vi "Add Error Core.vi"(8 "error in (no error)":errorcluster, 10 "String to Append":string, 11 "Error":T1) -> (0 "error out":errorcluster)   [LabVIEW 2021, in "CIFCoreCommon.lvlib"]
uses:
  CIFCoreCommon.lvlib
  <vilib>/CIF Foundation/CIF Utilities/Errors/Errors_CIF_U.lvlib
  Typedef/Errors.ctl
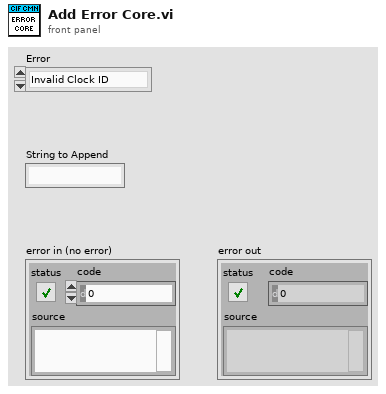
[diagram p1: front panel]
types:
  T1 = typedef "CIFCoreCommon.lvlib/Errors.ctl" = enum16{"Invalid Clock ID", "Long Sleep", "gRPC Server Not Found", "Config Parse", "Timestamp Wrap", "Delayed Execution", "Duplicate Channel", "Missing Channel", "Incorrect Type", "Flatten Error", "Unflatten Data", "Unique Name", "Plugin Not Found", "Plugin Type Not Found", "Plugin Version Not Found", "Manager Not Found", "Numerical Issue", "Time Jump", "Clock ID Match", "Channel Length", "Plugin Connection", "gRPC Server Connection", "PPL Name Match", "Build", "Config Log Parse", "Plugin Load", "UI Subpanel Load", "Python Name", "Invalid Name", "Unable to Change Ch Buffer", "Failed Kill", "Failed SysExec", "Function Not Implemented", "Load Timeout", "Invalid FTE", "Manager Crash"}
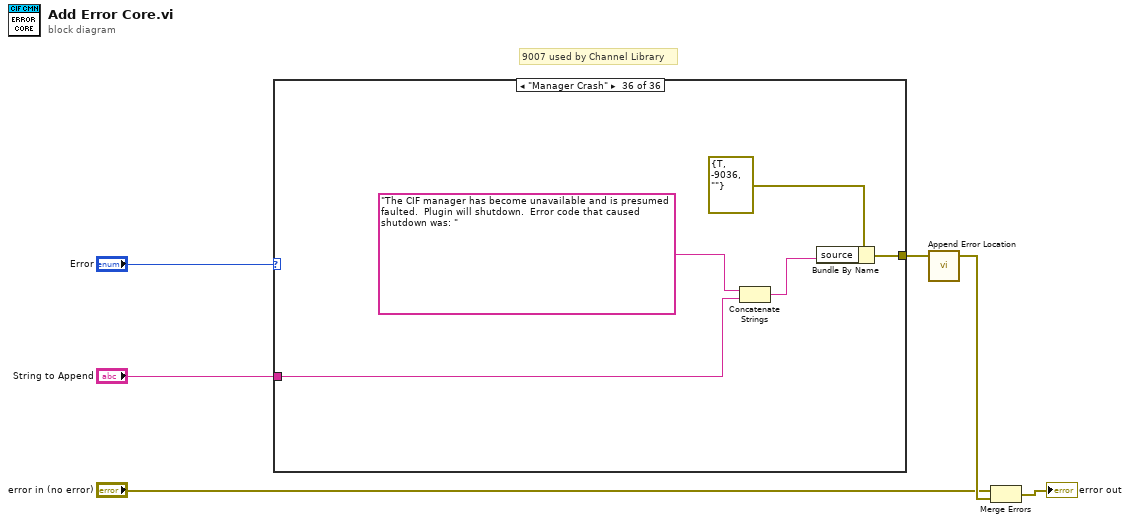
[diagram p0: block diagram]
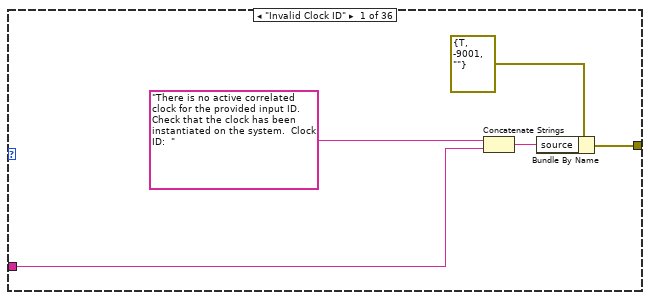
[diagram p2: hidden frame]
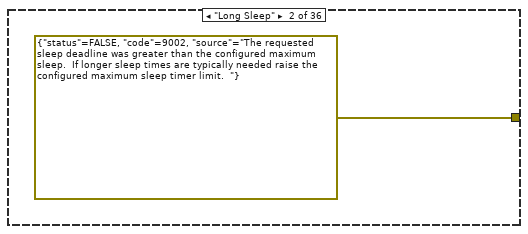
[diagram p3: hidden frame]
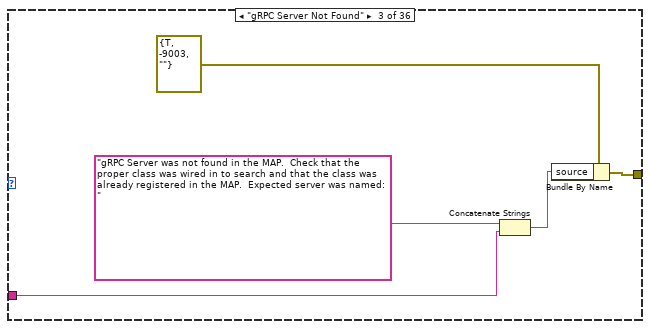
[diagram p4: hidden frame]
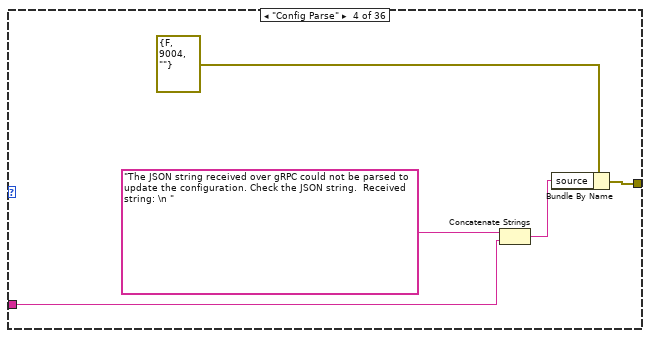
[diagram p5: hidden frame]
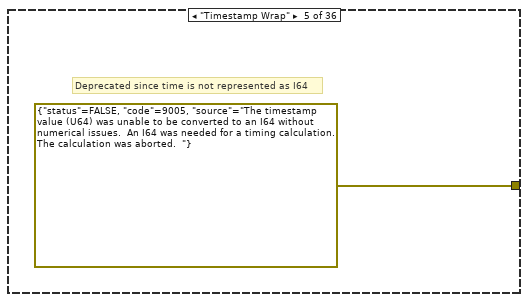
[diagram p6: hidden frame]
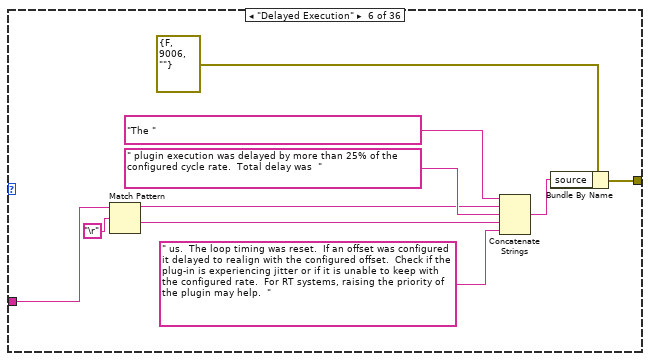
[diagram p7: hidden frame]
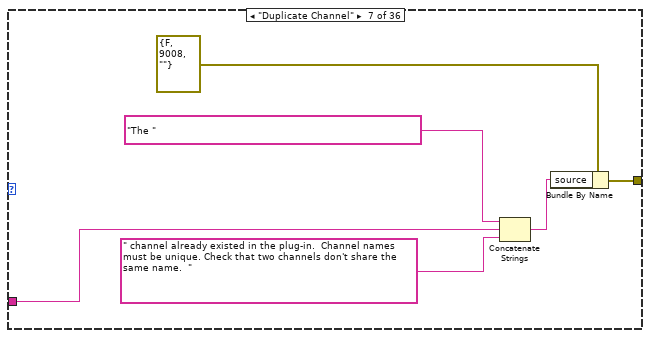
[diagram p8: hidden frame]
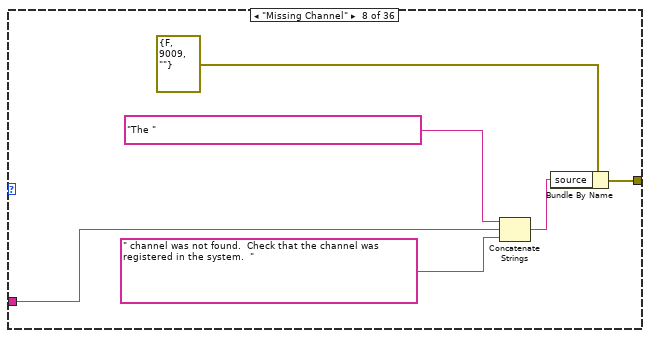
[diagram p9: hidden frame]
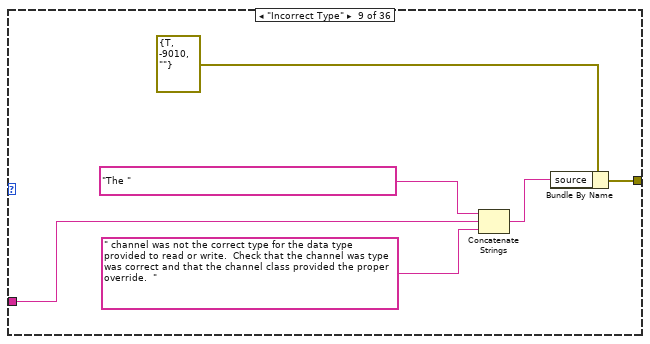
[diagram p10: hidden frame]
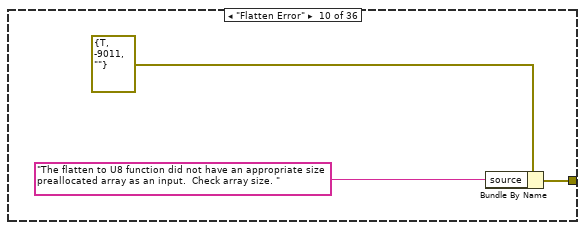
[diagram p11: hidden frame]
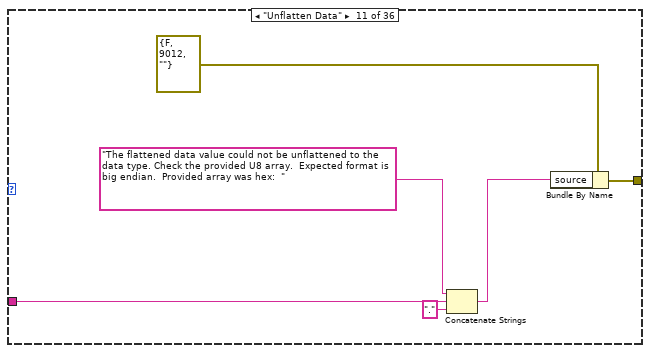
[diagram p12: hidden frame]
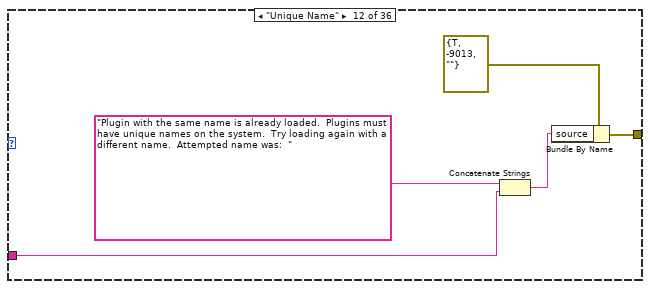
[diagram p13: hidden frame]
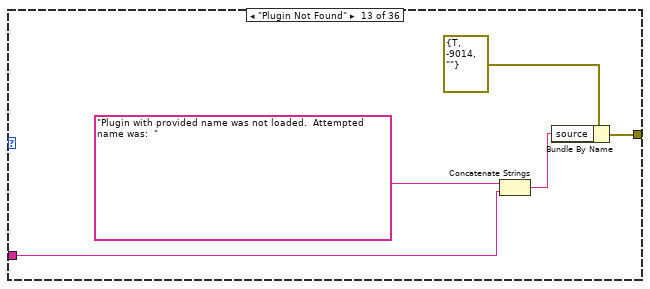
[diagram p14: hidden frame]
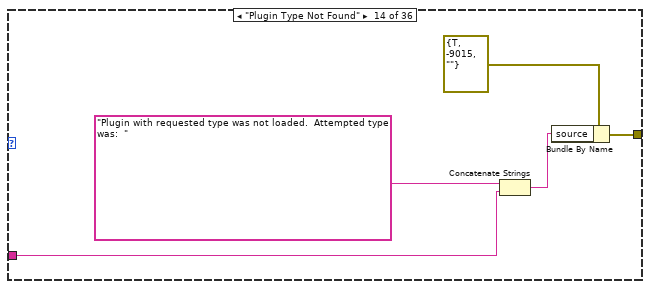
[diagram p15: hidden frame]
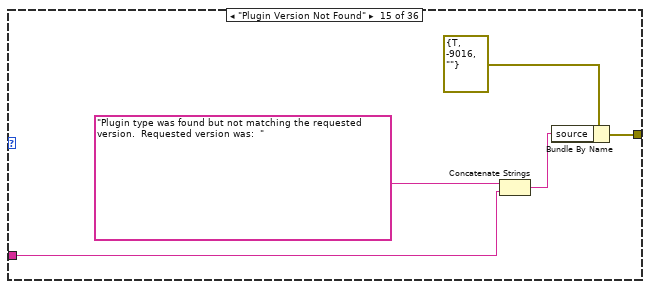
[diagram p16: hidden frame]
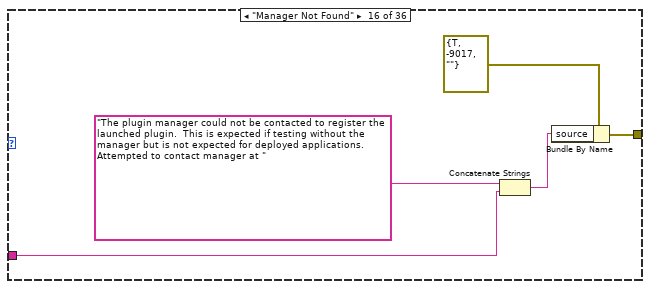
[diagram p17: hidden frame]
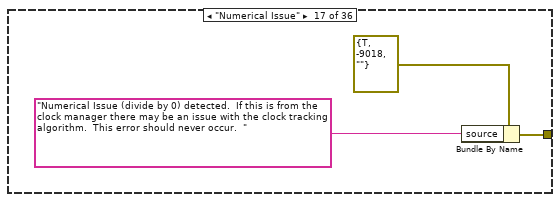
[diagram p18: hidden frame]
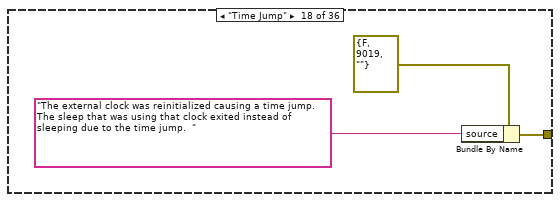
[diagram p19: hidden frame]
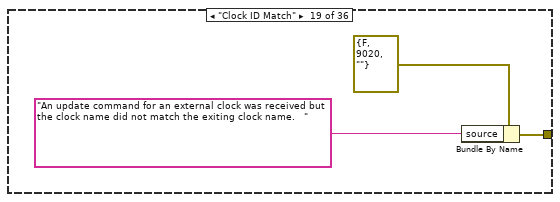
[diagram p20: hidden frame]
diagram:
  # "9007 used by Channel Library"
  n1 = case shown="\"Manager Crash\"" "Error" {
    tunnel: "String to Append" -> [w8 _ w14 w19 _ w28 w36 w40 w46 _ w57 w62 w67 w72 w77 w82 _ _ _ _ w98 w103 w108 w113 w118 _ _ w129 w134 _ w143 w148 w153 w158 w163 w167]
    tunnel: [w10 errorcluster {"status"=FALSE, "code"=9002, "source"="The requested sleep deadline was greater than the configured maximum sleep.  If longer sleep times are typically needed raise the configured maximum sleep timer limit.  "} ("Invalid ID") w16 w21 errorcluster {"status"=FALSE, "code"=9005, "source"="The timestamp value (U64) was unable to be converted to an I64 without numerical issues.  An I64 was needed for a timing calculation.  The calculation was aborted.  "} ("Invalid ID") w32 w38 w44 w50 w53 w59 w64 w69 w74 w79 w84 w87 w90 w93 w96 w101 w106 w111 w116 w121 w124 w127 w132 w137 w140 w145 w150 w155 w160 w165 w170] -> w5
    frame "Invalid Clock ID" {
      n2 = Concatenate Strings("There is no active correlated clock for the provided input ID.  Check that the clock has been instantiated on the system.  Clock ID:  " ("source"), w8) -> (w7:string)
      n3 = Bundle By Name(cluster=errorcluster {"status"=TRUE, "code"=-9001, "source"=""} ("Invalid ID"), "source"=w7) -> (w10:errorcluster)
    }
    frame "Long Sleep" {
    }
    frame "gRPC Server Not Found" {
      n4 = Concatenate Strings("gRPC Server was not found in the MAP.  Check that the proper class was wired in to search and that the class was already registered in the MAP.  Expected server was named:  " ("source"), w14) -> (w15:string)
      n5 = Bundle By Name(cluster=errorcluster {"status"=TRUE, "code"=-9003, "source"=""} ("Invalid ID"), "source"=w15) -> (w16:errorcluster)
    }
    frame "Config Parse" {
      n6 = Concatenate Strings("The JSON string received over gRPC could not be parsed to update the configuration. Check the JSON string.  Received string: \n " ("source"), w19) -> (w20:string)
      n7 = Bundle By Name(cluster=errorcluster {"status"=FALSE, "code"=9004, "source"=""} ("Invalid ID"), "source"=w20) -> (w21:errorcluster)
    }
    frame "Timestamp Wrap" {
      # "Deprecated since time is not represented as I64"
    }
    frame "Delayed Execution" {
      n8 = Match Pattern(string=w28, regular expression="\r") -> (before substring=w27:string, after substring=w25:string)  [unwired: 1 in, 2 out]
      n9 = Concatenate Strings("The " ("source"), w27, " plugin execution was delayed by more than 25% of the configured cycle rate.  Total delay was  " ("source"), w25, " us.  The loop timing was reset.  If an offset was configured it delayed to realign with the configured offset.  Check if the plug-in is experiencing jitter or if it is unable to keep with the configured rate.  For RT systems, raising the priority of the plugin may help.  " ("source")) -> (w31:string)
      n10 = Bundle By Name(cluster=errorcluster {"status"=FALSE, "code"=9006, "source"=""} ("Invalid ID"), "source"=w31) -> (w32:errorcluster)
    }
    frame "Duplicate Channel" {
      n11 = Concatenate Strings("The " ("source"), w36, " channel already existed in the plug-in.  Channel names must be unique. Check that two channels don't share the same name.  " ("source")) -> (w37:string)
      n12 = Bundle By Name(cluster=errorcluster {"status"=FALSE, "code"=9008, "source"=""} ("Invalid ID"), "source"=w37) -> (w38:errorcluster)
    }
    frame "Missing Channel" {
      n13 = Concatenate Strings("The " ("source"), w40, " channel was not found.  Check that the channel was registered in the system.  " ("source")) -> (w43:string)
      n14 = Bundle By Name(cluster=errorcluster {"status"=FALSE, "code"=9009, "source"=""} ("Invalid ID"), "source"=w43) -> (w44:errorcluster)
    }
    frame "Incorrect Type" {
      n15 = Concatenate Strings("The " ("source"), w46, " channel was not the correct type for the data type provided to read or write.  Check that the channel was type was correct and that the channel class provided the proper override.  " ("source")) -> (w47:string)
      n16 = Bundle By Name(cluster=errorcluster {"status"=TRUE, "code"=-9010, "source"=""} ("Invalid ID"), "source"=w47) -> (w50:errorcluster)
    }
    frame "Flatten Error" {
      n17 = Bundle By Name(cluster=errorcluster {"status"=TRUE, "code"=-9011, "source"=""} ("Invalid ID"), "source"="The flatten to U8 function did not have an appropriate size preallocated array as an input.  Check array size. ") -> (w53:errorcluster)
    }
    frame "Unflatten Data" {
      n18 = Concatenate Strings("The flattened data value could not be unflattened to the data type. Check the provided U8 array.  Expected format is big endian.  Provided array was hex:  " ("source"), w57, "." ("string")) -> (w55:string)
      n19 = Bundle By Name(cluster=errorcluster {"status"=FALSE, "code"=9012, "source"=""} ("Invalid ID"), "source"=w55) -> (w59:errorcluster)
    }
    frame "Unique Name" {
      n20 = Concatenate Strings("Plugin with the same name is already loaded.  Plugins must have unique names on the system.  Try loading again with a different name.  Attempted name was:  " ("source"), w62) -> (w63:string)
      n21 = Bundle By Name(cluster=errorcluster {"status"=TRUE, "code"=-9013, "source"=""} ("Invalid ID"), "source"=w63) -> (w64:errorcluster)
    }
    frame "Plugin Not Found" {
      n22 = Concatenate Strings("Plugin with provided name was not loaded.  Attempted name was:  " ("source"), w67) -> (w68:string)
      n23 = Bundle By Name(cluster=errorcluster {"status"=TRUE, "code"=-9014, "source"=""} ("Invalid ID"), "source"=w68) -> (w69:errorcluster)
    }
    frame "Plugin Type Not Found" {
      n24 = Concatenate Strings("Plugin with requested type was not loaded.  Attempted type was:  " ("source"), w72) -> (w73:string)
      n25 = Bundle By Name(cluster=errorcluster {"status"=TRUE, "code"=-9015, "source"=""} ("Invalid ID"), "source"=w73) -> (w74:errorcluster)
    }
    frame "Plugin Version Not Found" {
      n26 = Concatenate Strings("Plugin type was found but not matching the requested version.  Requested version was:  " ("source"), w77) -> (w78:string)
      n27 = Bundle By Name(cluster=errorcluster {"status"=TRUE, "code"=-9016, "source"=""} ("Invalid ID"), "source"=w78) -> (w79:errorcluster)
    }
    frame "Manager Not Found" {
      n28 = Concatenate Strings("The plugin manager could not be contacted to register the launched plugin.  This is expected if testing without the manager but is not expected for deployed applications.  Attempted to contact manager at " ("source"), w82) -> (w83:string)
      n29 = Bundle By Name(cluster=errorcluster {"status"=TRUE, "code"=-9017, "source"=""} ("Invalid ID"), "source"=w83) -> (w84:errorcluster)
    }
    frame "Numerical Issue" {
      n30 = Bundle By Name(cluster=errorcluster {"status"=TRUE, "code"=-9018, "source"=""} ("Invalid ID"), "source"="Numerical Issue (divide by 0) detected.  If this is from the clock manager there may be an issue with the clock tracking algorithm.  This error should never occur.  ") -> (w87:errorcluster)
    }
    frame "Time Jump" {
      n31 = Bundle By Name(cluster=errorcluster {"status"=FALSE, "code"=9019, "source"=""} ("Invalid ID"), "source"="The external clock was reinitialized causing a time jump.  The sleep that was using that clock exited instead of sleeping due to the time jump.  ") -> (w90:errorcluster)
    }
    frame "Clock ID Match" {
      n32 = Bundle By Name(cluster=errorcluster {"status"=FALSE, "code"=9020, "source"=""} ("Invalid ID"), "source"="An update command for an external clock was received but the clock name did not match the exiting clock name.   ") -> (w93:errorcluster)
    }
    frame "Channel Length" {
      n33 = Bundle By Name(cluster=errorcluster {"status"=TRUE, "code"=-9021, "source"=""} ("Invalid ID"), "source"="The internal length of the channel was incorrect.  The length should be set automatically so this is a developer error.  ") -> (w96:errorcluster)
    }
    frame "Plugin Connection" {
      n34 = Concatenate Strings("The plugin could not be found to complete the operation.  The requested plugin was: " ("source"), w98) -> (w99:string)
      n35 = Bundle By Name(cluster=errorcluster {"status"=TRUE, "code"=-9022, "source"=""} ("Invalid ID"), "source"=w99) -> (w101:errorcluster)
    }
    frame "gRPC Server Connection" {
      n36 = Concatenate Strings("The gRPC Server could not be connected.  The attempted address was: " ("source"), w103) -> (w104:string)
      n37 = Bundle By Name(cluster=errorcluster {"status"=TRUE, "code"=-9023, "source"=""} ("Invalid ID"), "source"=w104) -> (w106:errorcluster)
    }
    frame "PPL Name Match" {
      n38 = Concatenate Strings("Build was aborted to fix configuration.  The PPL name did not match the name of the build project or the version of the library did not match.  For UI builds, Instrument Studio requires the name of the PPL match the project.   The name and version were automatically updated.  It should build if you execute the build again.  " ("source"), w108) -> (w109:string)
      n39 = Bundle By Name(cluster=errorcluster {"status"=TRUE, "code"=-9024, "source"=""} ("Invalid ID"), "source"=w109) -> (w111:errorcluster)
    }
    frame "Build" {
      n40 = Concatenate Strings("Build was aborted to due to a parsing error in the pre or post build action.  It may be possible to remove the pre/post-build steps and manually perform pre/post build scripting steps.  " ("source"), w113) -> (w114:string)
      n41 = Bundle By Name(cluster=errorcluster {"status"=TRUE, "code"=-9025, "source"=""} ("Invalid ID"), "source"=w114) -> (w116:errorcluster)
    }
    frame "Config Log Parse" {
      n42 = Concatenate Strings("Config log file could not be parsed to created automated orchestration code.  Issue with line: " ("source"), w118) -> (w119:string)
      n43 = Bundle By Name(cluster=errorcluster {"status"=FALSE, "code"=9026, "source"=""} ("Invalid ID"), "source"=w119) -> (w121:errorcluster)
    }
    frame "Plugin Load" {
      # "Existing error code reused.  Message updated."
      n44 = Bundle By Name(cluster=errorcluster {"status"=TRUE, "code"=1003, "source"=""} ("Invalid ID"), "source"="The built plugin could not be loaded on the system by LabVIEW.  This can be caused by a missing dependency on the system (missing dll/so or called PPL) or by a malleable vi (vim) used on a LabVIEW Class wire (limitation of LabVIEW classes built as PPLs).  Recommended debug steps.  Assure the plugin code will run in interactive/debug mode.  Build sub-sections of the plugin until you can identify the parts that cause built PPLs to not load.  Check for debugging/benchmarking where the \"Get Timestamp.vim\" was used to make sure it is not on a Class wire.   ") -> (w124:errorcluster)
    }
    frame "UI Subpanel Load" {
      n45 = Bundle By Name(cluster=errorcluster {"status"=TRUE, "code"=-9027, "source"=""} ("Invalid ID"), "source"="The UI subpanels could not be loaded on the system.  This is normally due to an incorrect installation.  The subpanels are loaded dynamically from a built PPL.  The subpanel library (CIF Manager UI.x.x.x.lvlibp) is expected at <default CIF directory>\\PluginUI.  On Windows this is C:\\Users\\Public\\Documents\\CIF\\PluginUI.  Recommended debug steps.  Check that the file and directory exist and if needed repair installation.    ") -> (w127:errorcluster)
    }
    frame "Python Name" {
      n46 = Concatenate Strings("The name is not a valid Python variable name.  To facilitate Python orchestration it is recommended to change the name to:  " ("source"), w129) -> (w130:string)
      n47 = Bundle By Name(cluster=errorcluster {"status"=FALSE, "code"=9028, "source"=""} ("Invalid ID"), "source"=w130) -> (w132:errorcluster)
    }
    frame "Invalid Name" {
      n48 = Concatenate Strings("The name is not a valid.  The attempted name was:  " ("source"), w134) -> (w135:string)
      n49 = Bundle By Name(cluster=errorcluster {"status"=TRUE, "code"=-9029, "source"=""} ("Invalid ID"), "source"=w135) -> (w137:errorcluster)
    }
    frame "Unable to Change Ch Buffer" {
      n50 = Bundle By Name(cluster=errorcluster {"status"=FALSE, "code"=9030, "source"=""} ("Invalid ID"), "source"="A request to change the channel buffer size was made but a subscriber is already connected or the plugin is executing so the size cannot be changed.  Buffer size changes must be made when the plugin is not executing and no subcribers are connected to the FIFO channel.  ") -> (w140:errorcluster)
    }
    frame "Failed Kill" {
      n51 = Concatenate Strings("Failed to kill.  The command and response were:" ("source"), w143) -> (w142:string)
      n52 = Bundle By Name(cluster=errorcluster {"status"=FALSE, "code"=9031, "source"=""} ("Invalid ID"), "source"=w142) -> (w145:errorcluster)
    }
    frame "Failed SysExec" {
      n53 = Concatenate Strings("Failed call to sys exec. The command, error, and response were:" ("source"), w148) -> (w147:string)
      n54 = Bundle By Name(cluster=errorcluster {"status"=TRUE, "code"=-9032, "source"=""} ("Invalid ID"), "source"=w147) -> (w150:errorcluster)
    }
    frame "Function Not Implemented" {
      n55 = Concatenate Strings("The requested function has not been implemented.  Requested function was: " ("source"), w153) -> (w152:string)
      n56 = Bundle By Name(cluster=errorcluster {"status"=TRUE, "code"=-9033, "source"=""} ("Invalid ID"), "source"=w152) -> (w155:errorcluster)
    }
    frame "Load Timeout" {
      n57 = Concatenate Strings("The operation to load an external component timed out.  Component and requestor details were: " ("source"), w158) -> (w157:string)
      n58 = Bundle By Name(cluster=errorcluster {"status"=TRUE, "code"=-9034, "source"=""} ("Invalid ID"), "source"=w157) -> (w160:errorcluster)
    }
    frame "Invalid FTE" {
      n59 = Concatenate Strings("The future time event provided was out of range.  The provided FTE and system time were: " ("source"), w163) -> (w162:string)
      n60 = Bundle By Name(cluster=errorcluster {"status"=FALSE, "code"=9035, "source"=""} ("Invalid ID"), "source"=w162) -> (w165:errorcluster)
    }
    frame "Manager Crash" {
      n61 = Concatenate Strings("The CIF manager has become unavailable and is presumed faulted.  Plugin will shutdown.  Error code that caused shutdown was: " ("source"), w167) -> (w168:string)
      n62 = Bundle By Name(cluster=errorcluster {"status"=TRUE, "code"=-9036, "source"=""} ("Invalid ID"), "source"=w168) -> (w170:errorcluster)
    }
  }
  n63 = call <vilib>:"Append Error Location.vi"("error in (no error)"=w5) -> ("error out"=w6:errorcluster)  [unwired: 4 in]
  n64 = Merge Errors("error in (no error)", w6) -> (→"error out":errorcluster)
